vi "Node_Init.vi"(0 "object in":refnum<class "Node.lvclass">, 2 "Value":dbl, 5 "Error In":errorcluster) -> (14 "object out":refnum<class "Node.lvclass">, 19 "Error Out":errorcluster)   [LabVIEW 2024, in "Node.lvclass"]
uses:
  Node.lvclass
  Node.lvclass/Node.ctl
panel:
  # "Connector Pane"
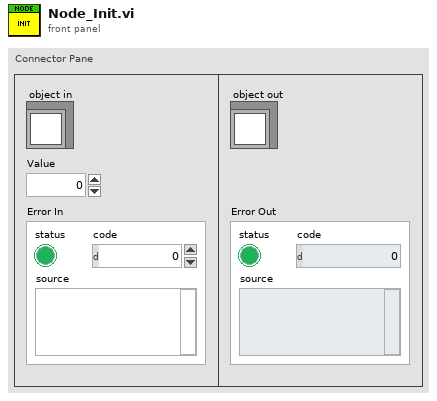
[diagram p1: front panel]
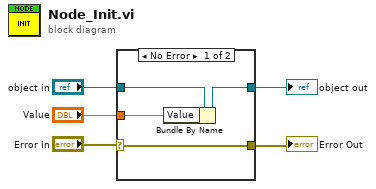
[diagram p0: block diagram]
diagram:
  n1 = case shown="No Error" "Error In" {
    selector: "Error In" -> [w7 w10]
    tunnel: "object in" -> [w9 w11]
    tunnel: [w8 w11] -> w4
    tunnel: [w7 w10] -> w2
    tunnel: "Value" -> [w6 _]
    frame No Error {
      n2 = Bundle By Name(cluster=w9, "Value"=w6) -> (w8:refnum<class "Node.lvclass">)
    }
    frame Error {
    }
  }
  "object out" <- w4
  "Error Out" <- w2
